vi "Error Handler - Event Handling Loop.vi"(8 "error in (no error)":errorcluster, 10 "Ignore Errors (Runtime)":i32[](array[numeric]), 11 "Message Queue":refnum<queue>) -> (0 "dup error in":errorcluster, 3 "dup Message Queue":refnum<queue>)   [LabVIEW 2020, in "SQSnobFit Control Panel.lvlib"]
doc: "Process an error that occurred in the Event Handling Loop, either by ignoring it, or generating an \"Error\" message."
uses:
  SQSnobFit Control Panel.lvlib
  support/Message Queue/Message Cluster.ctl
  support/Message Queue/Message Queue.lvlib
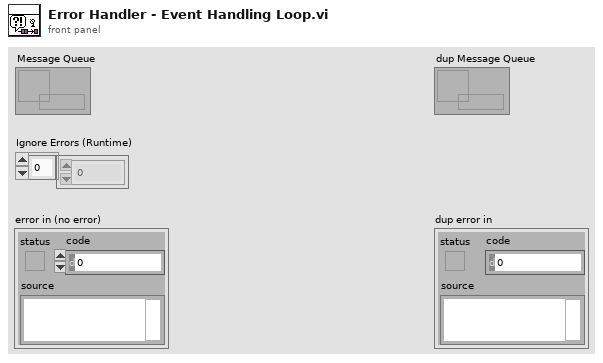
[diagram p1: front panel]
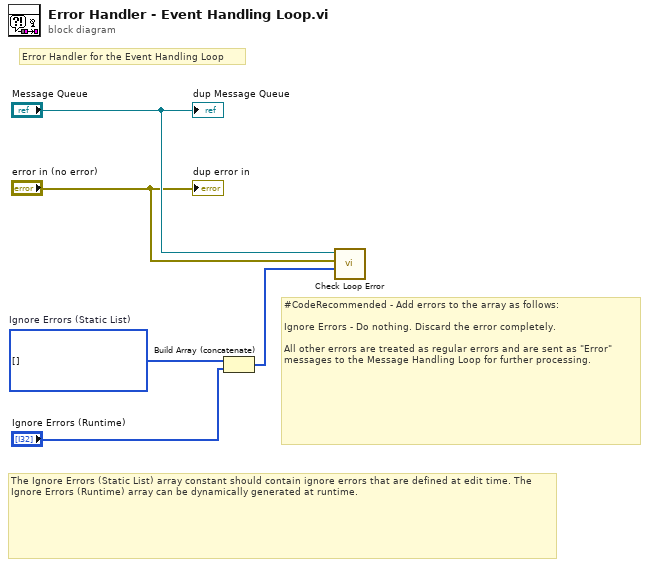
[diagram p0: block diagram]
diagram:
  w4 = i32[] []  # Ignore Errors (Static List)
  # "The Ignore Errors (Static List) array constant should contain ignore errors that are defined at edit time. The Ignore Errors (Runtime) array can be dynamically generated at runtime."
  # "#CodeRecommended - Add errors to the array as follows:\n\nIgnore Errors - Do nothing. Discard the error completely.\n\nAll other errors are treated as regular errors and are sent as \"Error\" messages to the Message Handling Loop for further processing."
  # "Error Handler for the Event Handling Loop"
  n1 = Build Array (concatenate)(w4, "Ignore Errors (Runtime)") -> (w3:i32[])
  n2 = call "Check Loop Error.vi"("Ignore Errors"=w3, "error to process"="error in (no error)", "Message Queue"="Message Queue") -> ()  [unwired: 7 in, 2 out]
  "dup Message Queue" <- "Message Queue"
  "dup error in" <- "error in (no error)"
